vi "User jsObject Array.vi"(7 "DB Connection Ref":T1, 8 "error in (no error)":errorcluster, 9 "USERS (empty)":T2[](array[typedef]), 10 "Users jsObject Array Name (\"USERS\")":string="USERS", 11 "Previous String (\"\")":string) -> (0 "error out":errorcluster, 2 "Users jsObject Array":string, 3 "User jsObject Definition":string)   [LabVIEW 2011]
uses:
  User Record.ctl
  Summitek EXT/ODBC/SQL Controls/Connection Refnum.ctl
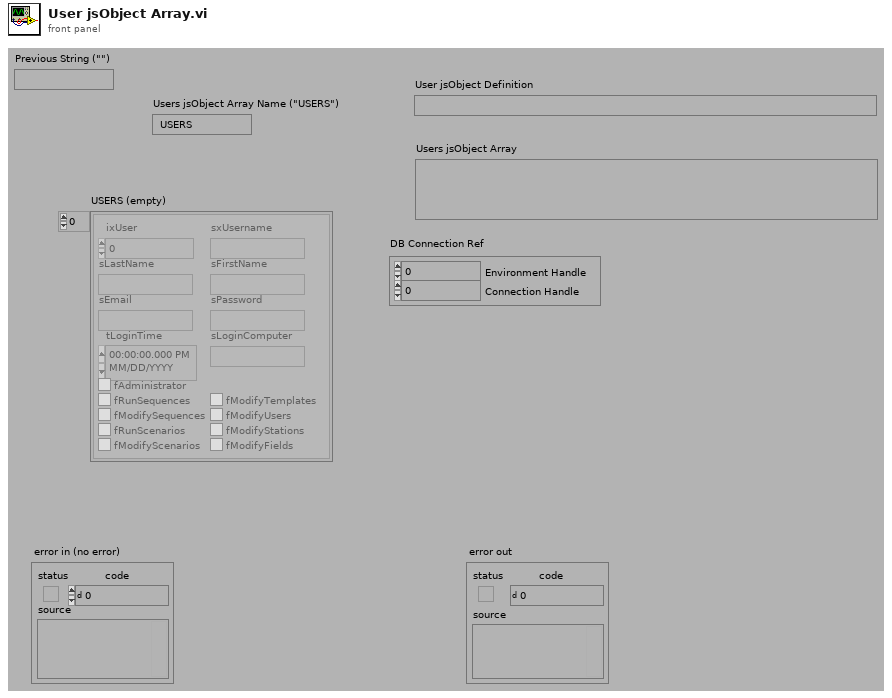
[diagram p1: front panel]
types:
  T1 = typedef "Connection Refnum.ctl" = cluster{"Environment Handle":i32, "Connection Handle":i32}
  T2 = typedef "User Record.ctl" = cluster{"ixUser":i32, "sxUsername":string, "sLastName":string, "sFirstName":string, "sEmail":string, "sPassword":string, "tLoginTime":timestamp, "sLoginComputer":string, "fAdministrator":bool, "fRunSequences":bool, "fModifySequences":bool, "fRunScenarios":bool, "fModifyScenarios":bool, "fModifyTemplates":bool, "fModifyUsers":bool, "fModifyStations":bool, "fModifyFields":bool}
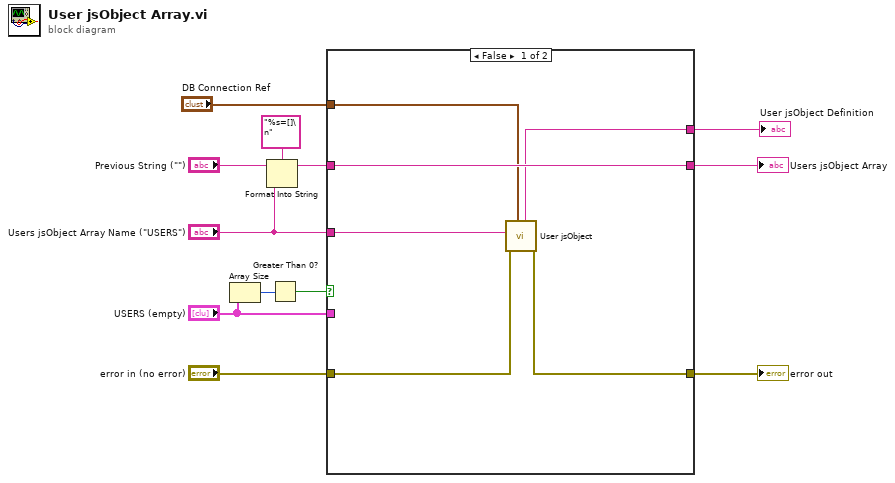
[diagram p0: block diagram]
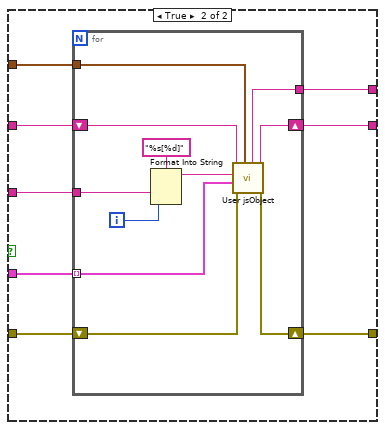
[diagram p2: hidden frame]
diagram:
  n1 = Array Size(array="USERS (empty)") -> (size(s)=w4:i32)
  n2 = Format Into String(format string="%s=[]\n", initial string="Previous String (\"\")", "Users jsObject Array Name (\"USERS\")") -> (resulting string=w8:string)  [unwired: 1 in, 1 out]
  n3 = Greater Than 0?(x=w4) -> (x > 0?=w3:bool)
  n4 = case shown="False" w3 {
    tunnel: [w18 w26] -> w12
    tunnel: "error in (no error)" -> [w17 w25]
    tunnel: [w16 w24] -> w10
    tunnel: w8 -> [w18 w23]
    tunnel: "Users jsObject Array Name (\"USERS\")" -> [w14 w22]
    tunnel: "USERS (empty)" -> [_ w21]
    tunnel: [w15 w20] -> w2
    tunnel: "DB Connection Ref" -> [w13 w19]
    frame False {
      n5 = call "User jsObject.vi"("DB Connection Ref"=w13, "error in (no error)"=w17, "User jsObject Name (\"USER\")"=w14) -> ("error out"=w16:errorcluster, "User jsObject Definition"=w15:string)  [unwired: 2 in, 5 out]
    }
    frame True {
      n6 = for {
        tunnel: w21 -> [w34] mode=indexing
        shift-right: [w35] -> w26
        shift-left: w23 -> [w37]
        shift-right: [w29] -> w24
        shift-left: w25 -> [w36]
        tunnel: w22 -> [w30]
        tunnel: [w28] -> w20
        tunnel: w19 -> [w27]
        i -> [w31]
        n7 = Format Into String(format string="%s[%d]", w30, w31) -> (resulting string=w32:string)  [unwired: 2 in, 1 out]
        n8 = call "User jsObject.vi"("DB Connection Ref"=w27, "error in (no error)"=w36, "User Record (empty)"=w34, "User jsObject Name (\"USER\")"=w32, "Previous String (\"\")"=w37) -> ("error out"=w29:errorcluster, "User jsObject"=w35:string, "User jsObject Definition"=w28:string)  [unwired: 4 out]
      }
    }
  }
  "Users jsObject Array" <- w12
  "error out" <- w10
  "User jsObject Definition" <- w2
